vi "Find State Data Cluster.vi"(8 "error in (no error)":errorcluster, 11 "QControl Class Refnum in":refnum<vi>) -> (0 "error out":errorcluster, 2 "State Data Cluster":refnum<vi>, 3 "QControl Class Refnum (dup)":refnum<vi>)   [LabVIEW 2015, in "State Accessor Scripter.lvclass"]
uses:
  State Accessor Scripter.lvclass
  <vilib>/ErrorRing/Error Ring.xnode
  <vilib>/Utility/error.llb/Error Cluster From Error Code.vi
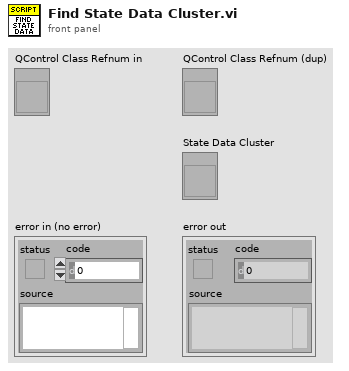
[diagram p1: front panel]
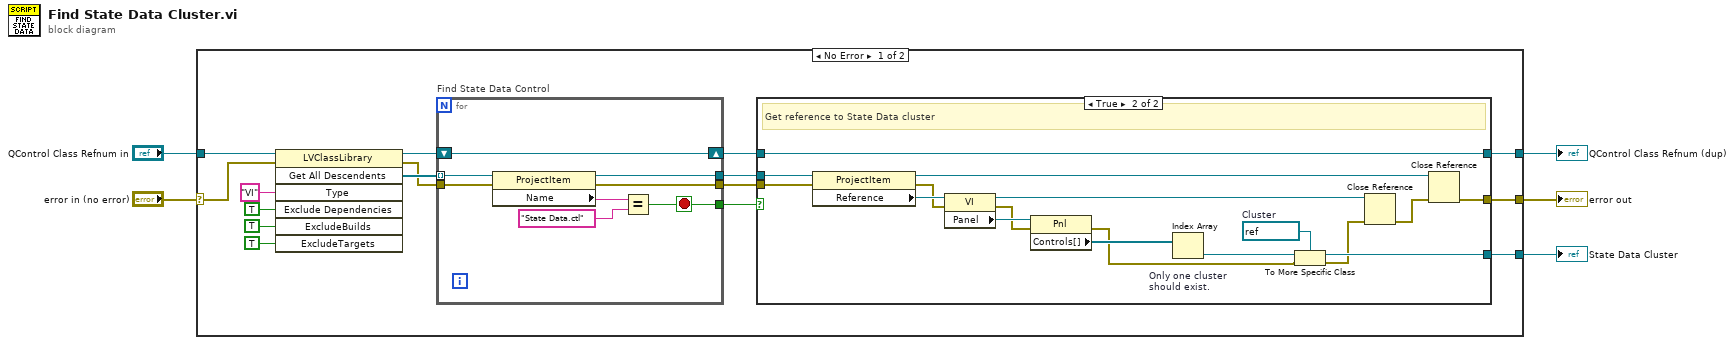
[diagram p0: block diagram]
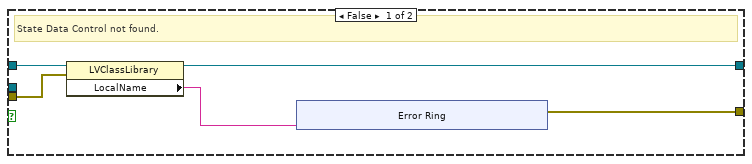
[diagram p2: hidden frame]
diagram:
  n1 = case shown="No Error" "error in (no error)" {
    selector: "error in (no error)" -> [w9 w60]
    tunnel: [w11 w60] -> w4
    tunnel: "QControl Class Refnum in" -> [w21 w59]
    tunnel: [w10 _] -> w3
    tunnel: [w6 w59] -> w1
    frame No Error {
      n2 = invoke class="LVClassLibrary" method="Get All Descendents"(reference=w21, error in=w9, "Type"="VI", "Exclude Dependencies"=TRUE ("ExcludeDependencies"), "ExcludeBuilds"=TRUE, "ExcludeTargets"=TRUE) -> (reference out=w8:refnum<vi>, error out=w15:errorcluster, "All Descendents"=w16:refnum<vi>[])  [unwired: 1 in, 4 out]
      n3 = for "Find State Data Control" {
        tunnel: w16 -> [w58] mode=indexing
        tunnel: [w55] -> w12
        tunnel: [w54] -> w14
        tunnel: w15 -> [w53]
        tunnel: [w52] -> w13
        shift-right: [w51] -> w7
        shift-left: w8 -> [w51]
        stop <- w54 stop-if-true
        n4 = property class="ProjectItem"(reference=w58, error in=w53) -> (reference out=w55:refnum<vi>, error out=w52:errorcluster, "Name"=w57:string)
        n5 = Equal?(x=w57, y="State Data.ctl") -> (x = y?=w54:bool)
      }
      n6 = case shown="True" w14 {
        tunnel: w13 -> [w25 w49]
        tunnel: w12 -> [_ w50]
        tunnel: [w22 w35] -> w11
        tunnel: [_ w43] -> w10
        tunnel: w7 -> [w26 w34]
        tunnel: [w24 w34] -> w6
        frame False {
          # "State Data Control not found."
          n7 = property class="LVClassLibrary"(reference=w26, error in=w25) -> (reference out=w24:refnum<vi>, "LocalName"=w23:string)  [unwired: 1 out]
          n8 = xnode "Error Ring"("parameter 0"=w23) -> ("error out"=w22:errorcluster)
        }
        frame True {
          w42 = refnum<vi> refnum  # Cluster
          # "Get reference to State Data cluster"
          n9 = property class="ProjectItem"(reference=w50, error in=w49) -> (reference out=w37:refnum<vi>, error out=w47:errorcluster, "Reference"=w48:refnum<vi>)
          n10 = property class="VI"(reference=w48, error in=w47) -> (reference out=w39:refnum<vi>, error out=w45:errorcluster, "Panel"=w46:refnum<vi>)
          n11 = property class="Pnl"(reference=w46, error in=w45) -> (error out=w41:errorcluster, "Controls[]"=w44:refnum<vi>[])  [unwired: 1 out]
          n12 = Index Array "Only one cluster \nshould exist."(array=w44) -> (element=w40:refnum<vi>)  [unwired: 1 in]
          n13 = To More Specific Class(target class=w42, reference=w40, error in=w41) -> (specific class reference=w43:refnum<vi>, error out=w38:errorcluster)
          n14 = Close Reference(reference=w39, error in (no error)=w38) -> (error out=w36:errorcluster)
          n15 = Close Reference(reference=w37, error in (no error)=w36) -> (error out=w35:errorcluster)
        }
      }
    }
    frame Error {
    }
  }
  "error out" <- w4
  "State Data Cluster" <- w3
  "QControl Class Refnum (dup)" <- w1
